vi "compress image to 65k_StateM.vi"(5 "Image":T1, 7 "error in (no error)":errorcluster) -> (0 "Data String":string, 3 "error out":errorcluster)   [LabVIEW 2011]
uses:
  IMAQ Image.ctl
  nivision.dll
  NI_Vision_Development_Module.lvlib
  C:/Program Files/National Instruments/LabVIEW 2011/resource/objmgr/IMAQImage.rc
panel:
  out "x*y":i32
  out "x/y":dbl(graph)
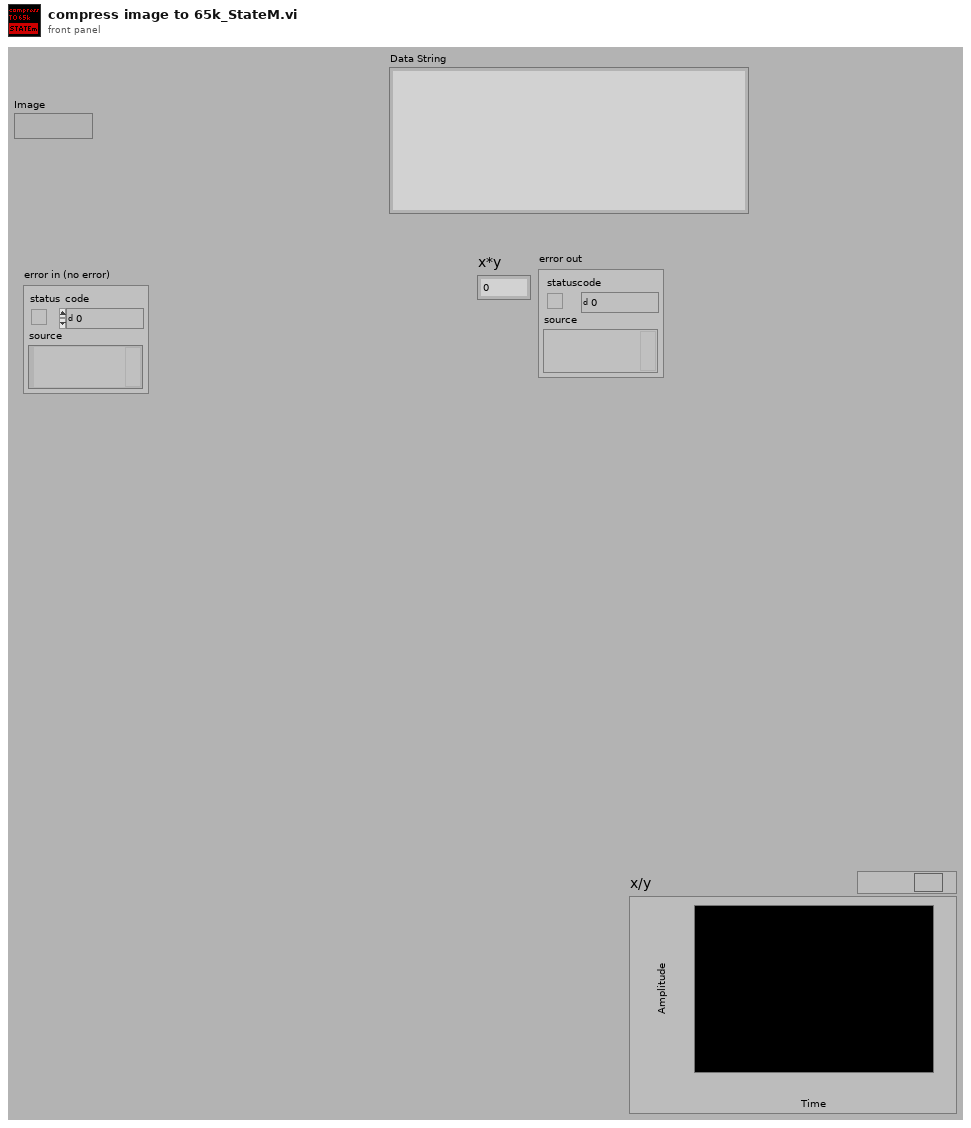
[diagram p1: front panel]
types:
  T1 = typedef "IMAQ Image.ctl" = refnum<image>
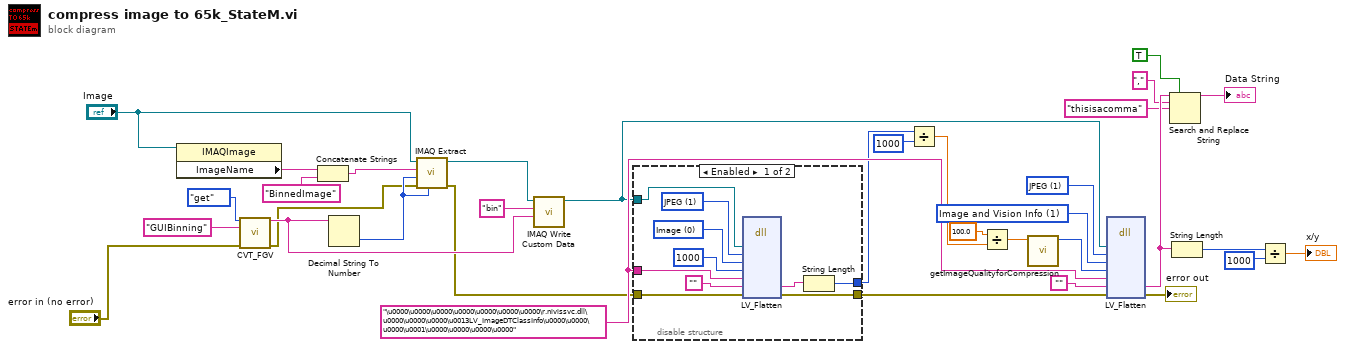
[diagram p0: block diagram]
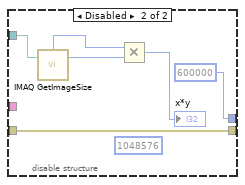
[diagram p2: hidden frame]
diagram:
  w23 = 1 items=["Image", "Image and Vision Info", "Reference to Image"] ("Type of Flatten (Image and Vision Info)")
  w22 = 1 items=["None", "JPEG", "PACKED BINARY"] ("Compression (None)")
  w25 = "\u0000\u0000\u0000\u0000\u0000\u0000\u0000\r.nivissvc.dll\u0000\u0000\u0000\u0013LV_ImageDTClassInfo\u0000\u0000\u0000\u0001\u0000\u0000\u0000\u0000" ("data string")
  n1 = property class="IMAQImage"(reference="Image") -> ("ImageName"=w6:string)  [unwired: 1 in, 2 out]
  n2 = call "CVT_FGV.vi"("command"=enum16{"set", "get", "reset", "get all"}."get", "variable"="GUIBinning" ("command or variable name"), "error in"="error in (no error)") -> ("value out"=w10:string, "error out"=w2:errorcluster)  [unwired: 10 in, 1 out]
  n3 = Concatenate Strings(w6, "BinnedImage" ("command or variable name")) -> (w4:string)
  n4 = Decimal String To Number(string=w10) -> (number=w12:i32)  [unwired: 2 in, 1 out]
  n5 = call "IMAQ Extract"("Y Step Size"=w12, "error in (no error)"=w2, "X Step Size"=w12, "Image Dst"=w4, "Image Src"="Image") -> ("error out"=w1:errorcluster, "Image Dst Out"=w9:T1)  [unwired: 5 in]
  n6 = call "IMAQ Write Custom Data"("Custom Data In"=w10, "Key"="bin", "Image"=w9) -> ("Image Out"=w8:T1)  [unwired: 7 in, 1 out]
  n7 = disable-structure shown="Enabled" {
    disable-tunnel: w8 -> [w44 w49]
    disable-tunnel: w1 -> [w43 w50]
    disable-tunnel: [w38 w50] -> w34
    disable-tunnel: w25 -> [w36 _]
    disable-tunnel: [w35 600000 ("Quality (750) 3")] -> w21
    frame Enabled {
      w41 = 0 items=["Image", "Image and Vision Info", "Reference to Image"] ("Type of Flatten (Image and Vision Info)")
      w42 = 1 items=["None", "JPEG", "PACKED BINARY"] ("Compression (None)")
      n8 = dll-call lib="nivision.*" fn="LV_Flatten"("Image"=w44, "compressionType"=w42, "flattenType"=w41, "quality"=1000 ("Quality (750) 3"), "data string"=w36, "output param"="", "error in (no error)"=w43) -> ("output param"=w37:string, "error in (no error)"=w38:errorcluster)  [unwired: 8 in, 3 out]
      n9 = String Length(string=w37) -> (length=w35:i32)
    }
    frame Disabled {
      (unwired) 1048576 ("x*y 2")
      n10 = call "IMAQ GetImageSize"("Image"=w49) -> ("Y Resolution"=w48:i32, "X Resolution"=w47:i32)  [unwired: 3 in, 1 out]
      n11 = Multiply(x=w47, y=w48) -> (x*y=→"x*y":i32)
    }
  }
  n12 = Divide(x=w21, y=1000) -> (x/y=w28:dbl)
  n13 = Divide(x=100.0 ("mean limit in kByte"), y=w28) -> (x/y=w27:dbl)
  n14 = call "getImageQualityforCompression.vi"("compression rate"=w27) -> ("quality"=w26:i16)  [unwired: 10 in]
  n15 = dll-call lib="nivision.*" fn="LV_Flatten"("Image"=w8, "compressionType"=w22, "flattenType"=w23, "quality"=w26, "data string"=w25, "output param"="", "error in (no error)"=w34) -> ("output param"=w19:string, "error in (no error)"=→"error out":errorcluster)  [unwired: 8 in, 3 out]
  n16 = Search and Replace String(replace all?=TRUE ("replace all? (F)"), input string=w19, search string=",", replace string="thisisacomma" ("replace string (\"\")")) -> (result string=→"Data String":string)  [unwired: 4 in, 3 out]
  n17 = String Length(string=w19) -> (length=w33:i32)
  n18 = Divide(x=w33, y=1000) -> (x/y=→"x/y":dbl)
